vi "registerTelemetry.vi"(8 "error in (no error)":errorcluster, 11 "SAL_Listener in":refnum<class "SAL_Listener.lvclass">) -> (0 "error out":errorcluster, 3 "SAL_Listener out":refnum<class "SAL_Listener.lvclass">)   [LabVIEW 2015, in "SAL_Listener.lvclass"]
uses:
  SAL_Listener.lvclass
  SAL_Listener.lvclass/SAL_Listener.ctl
  SALLV_domeADB/SALLV_domeADB.lvlib
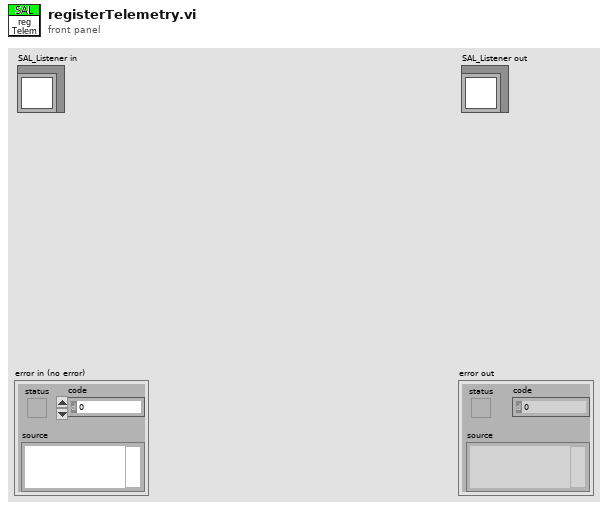
[diagram p1: front panel]
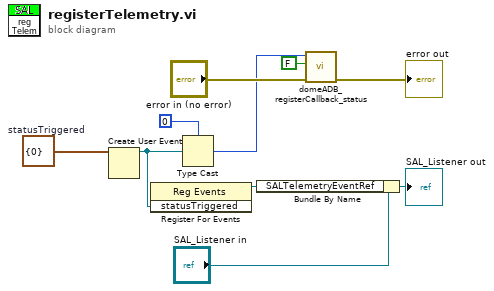
[diagram p0: block diagram]
diagram:
  w9 = cluster{"data":i32} {"data"=0}  # statusTriggered
  n1 = Create User Event(user event datatype=w9) -> (user event=w8:refnum<user-event>)  [unwired: 1 in, 1 out]
  n2 = register-events(w8) -> (reference out=w3:refnum<event-registration>)  [unwired: 2 in, 1 out]
  n3 = Type Cast(type=0, x=w8) -> (*(type *) &x=w6:i32)
  n4 = Bundle By Name(cluster="SAL_Listener in", "SALTelemetryEventRef"=w3) -> (→"SAL_Listener out":refnum<class "SAL_Listener.lvclass">)
  n5 = call "domeADB_registerCallback_status.vi"("error in (no error)"="error in (no error)", "skipOld"=FALSE, "handle"=w6) -> ("error out"=→"error out":errorcluster)  [unwired: 7 in, 1 out]
